vi "test14.2-MappingRelationshipByExternalRegistration_State.vi"() -> ()   [LabVIEW 2017, in "testcase-CSMBroadcast.lvclass"]
uses:
  testcase-CSMBroadcast.lvclass
  5f1321ef-d679-4204-8b32-271554a776bf.vi
  3afc563d-56e9-48a4-901d-19be23a22e68.vi
  src/user.lib/_NEVSTOP/Communicable State Machine(CSM)/AdvanceAPI/CSM - Revert Arguments-Safe String.vi
  src/user.lib/_NEVSTOP/Communicable State Machine(CSM)/AdvanceAPI/CSM - Make String Arguments Safe.vi
  src/user.lib/_NEVSTOP/Communicable State Machine(CSM)/AdvanceAPI/CSM - Break Down Multiple States String.vi
  src/user.lib/_NEVSTOP/Communicable State Machine(CSM)/AdvanceAPI/CSM - Keywords.vi
  src/user.lib/_NEVSTOP/Communicable State Machine(CSM)/_Polymophic/CSM - Replace Marks in Messages.vi
  src/user.lib/_NEVSTOP/Communicable State Machine(CSM)/_Shared/Trim Single-line Text.vi
  src/user.lib/_NEVSTOP/Communicable State Machine(CSM)/Communicable State Machine.lvlib
  <vilib>/addons/_JKI Toolkits/VI Tester/TestCase.llb/TestCase.lvclass
  CSM/CSM-Testcase.lvlib
  C:/Program Files (x86)/National Instruments/LabVIEW 2017/vi.lib/addons/_JKI Toolkits/VI Tester/TestCase.llb/TestCase.lvclass
panel:
  out "State History 2":string
  out "Loop Count":i32
  out "TestCase out":refnum<class "testcase-CSMBroadcast.lvclass">
  in  "TestCase in":refnum<class "testcase-CSMBroadcast.lvclass">
  out "error out":errorcluster
  in  "error in (no error)":errorcluster
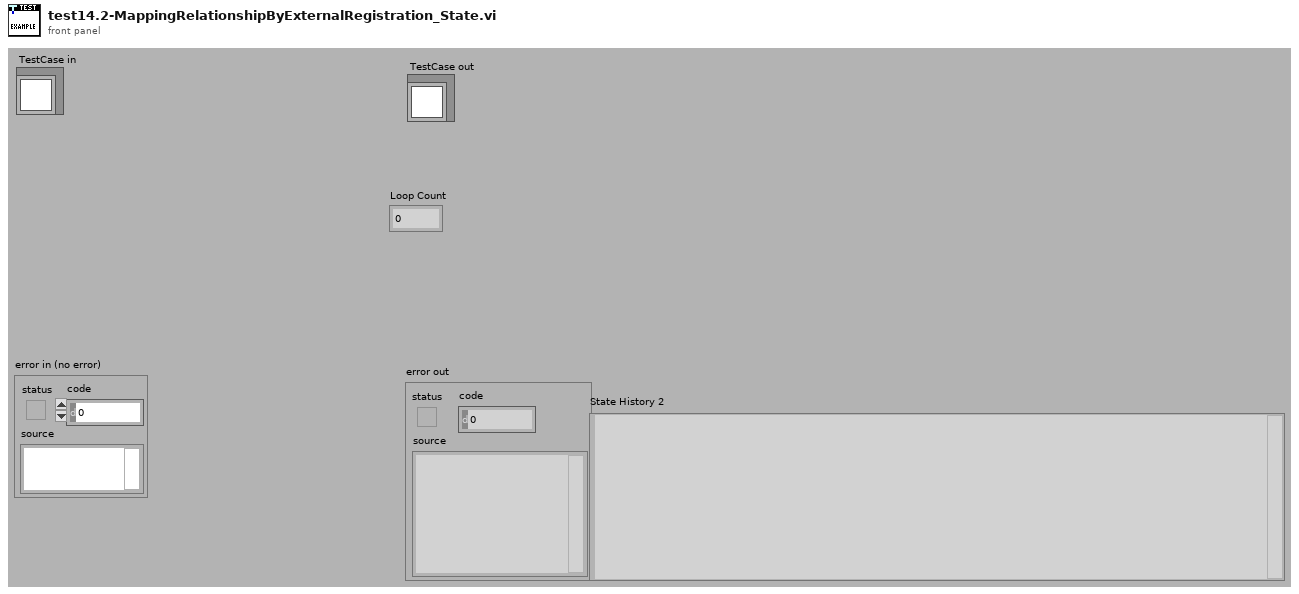
[diagram p1: front panel]
types:
  T1 = enum32{"Invalid", "Standard", "Closed", "Hidden", "Minimized", "Maximized"}
  T2 = enum32{"invalid app kind", "Development System", "Run Time System", "Student Edition", "Embedded LabVIEW", "Evaluation", "Custom"}
  T3 = cluster{"Status":string, "Source CSM":string, "Target CSM":string, "Target API":string}[]
  T4 = typedef "Communicable State Machine.lvlib/_CSM_Response Source Message.ctl" = cluster{"‘State":string, "’Arguments":string, "’Error":errorcluster}
  T5 = cluster{"Current VI Reference":refnum<vi>, "Close Panel on Exit?":bool}
  T6 = cluster{"Core":cluster{"Current VI Reference":refnum<vi>, "Close Panel on Exit?":bool}, "Your Boolean data":bool, "Your string data":string}
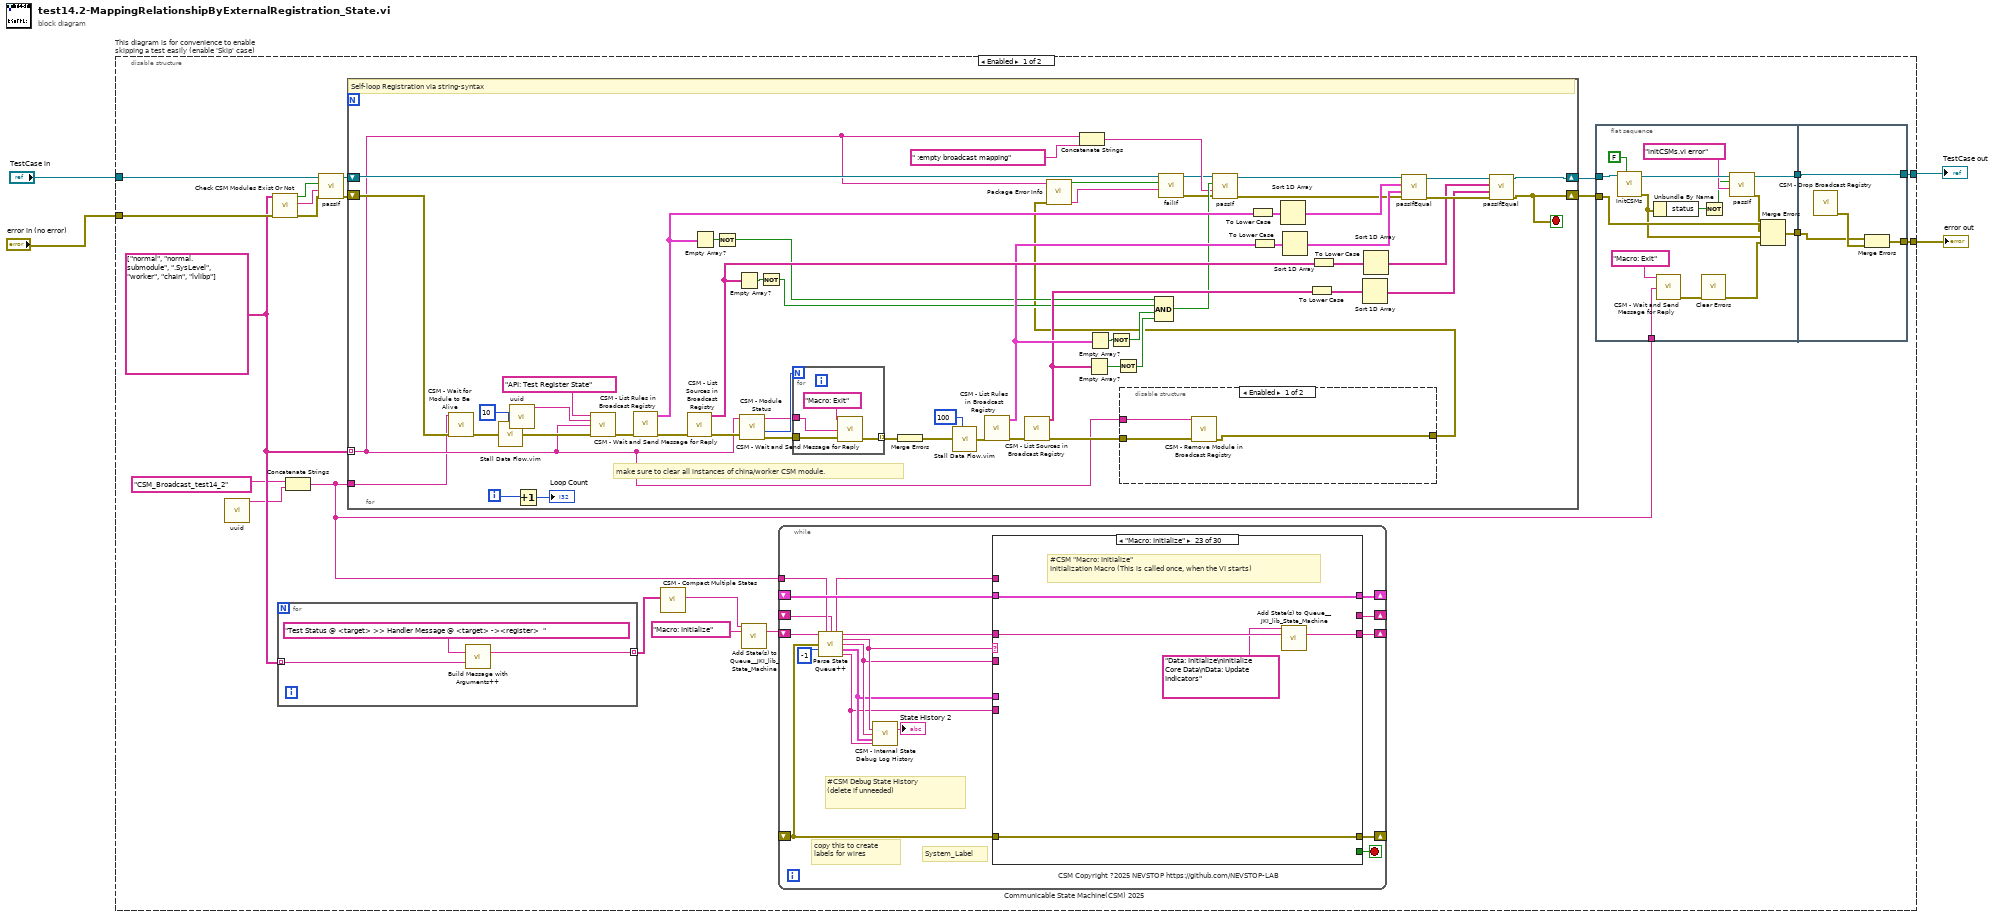
[diagram p0: block diagram]
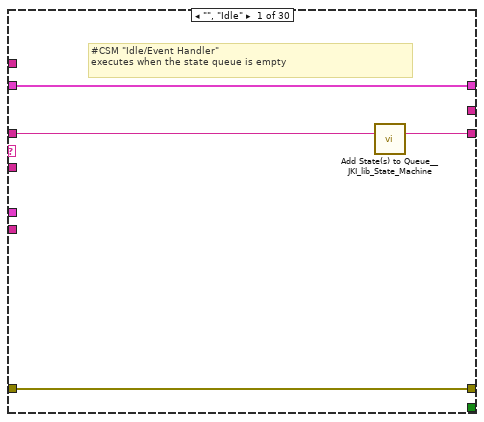
[diagram p2: hidden frame]
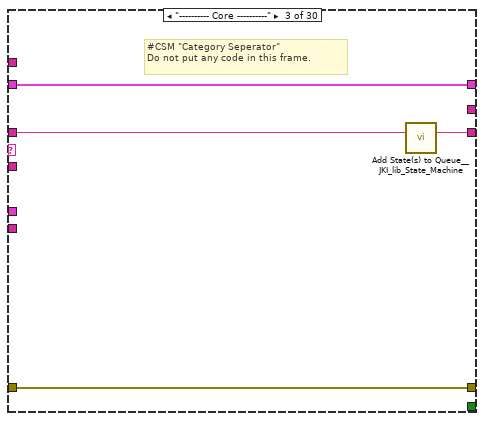
[diagram p4: hidden frame]
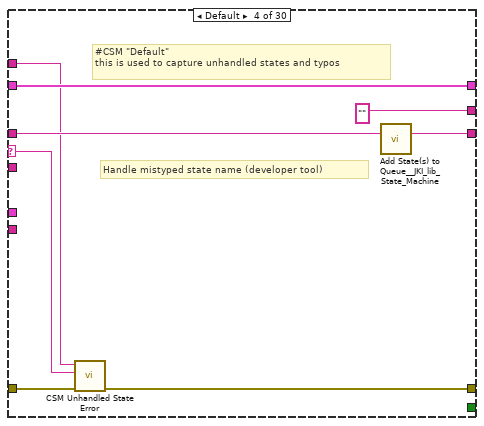
[diagram p5: hidden frame]
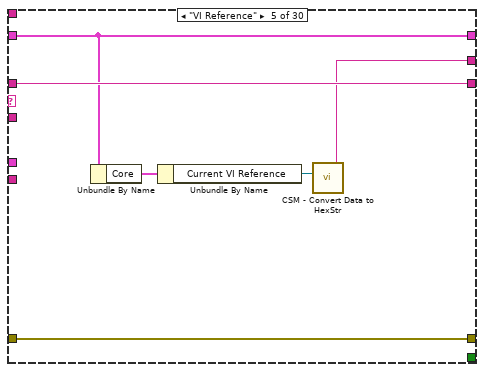
[diagram p6: hidden frame]
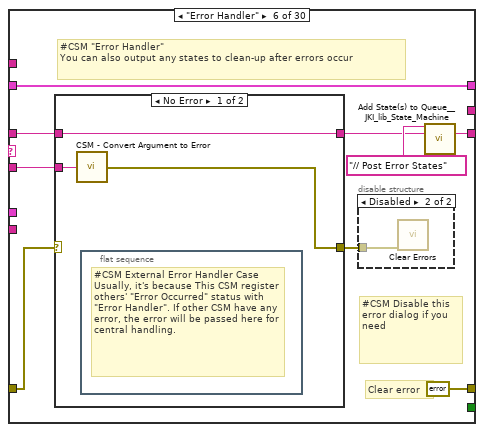
[diagram p7: hidden frame]
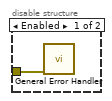
[diagram p8: hidden frame]
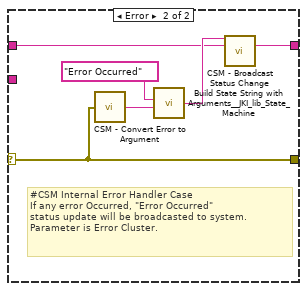
[diagram p9: hidden frame]
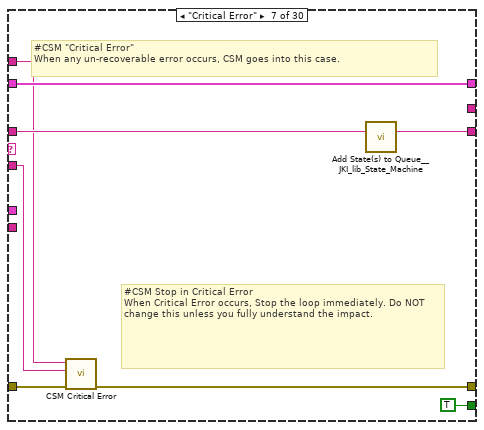
[diagram p10: hidden frame]
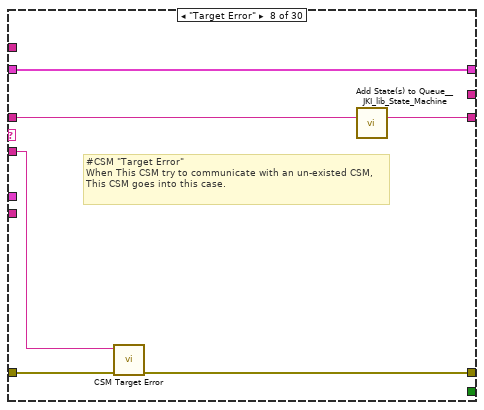
[diagram p11: hidden frame]
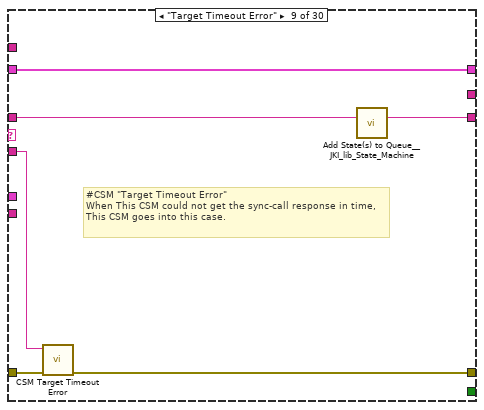
[diagram p12: hidden frame]
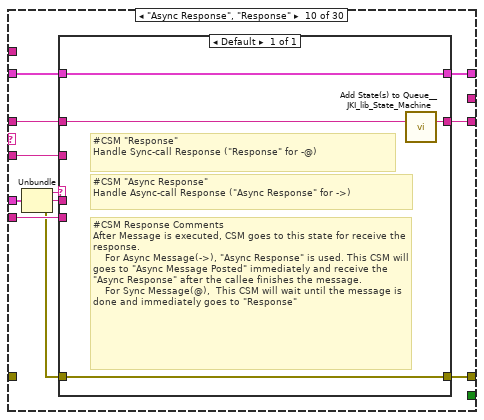
[diagram p13: hidden frame]
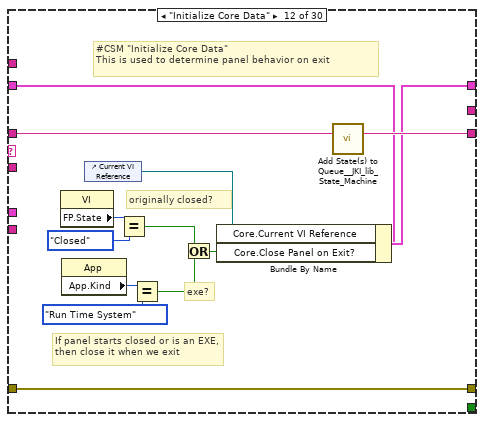
[diagram p15: hidden frame]
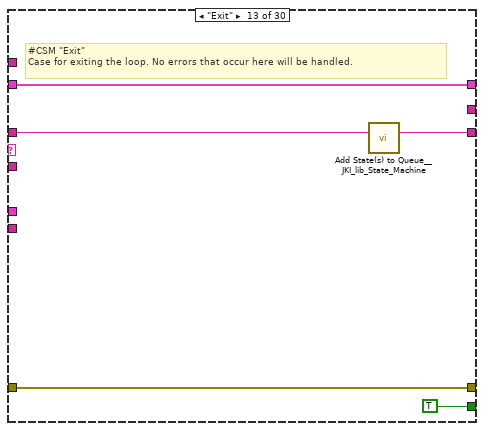
[diagram p16: hidden frame]
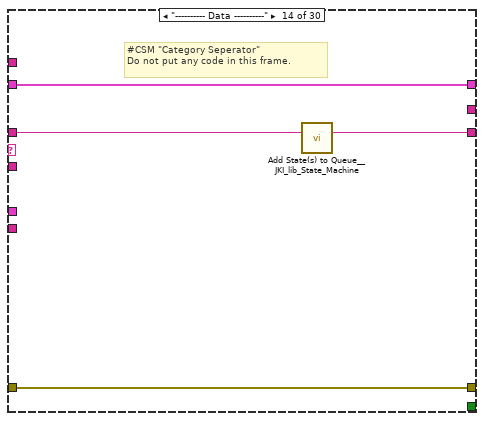
[diagram p17: hidden frame]
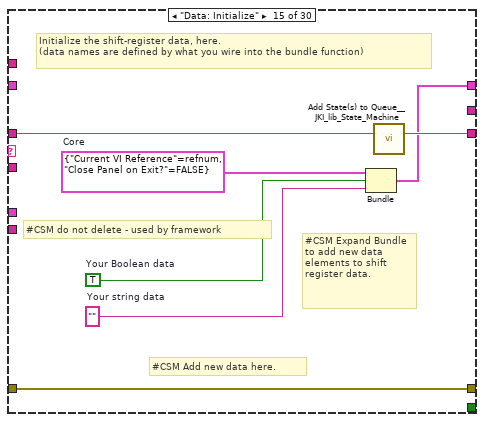
[diagram p18: hidden frame]
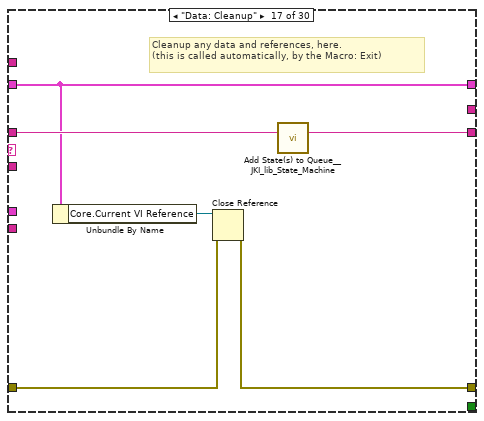
[diagram p20: hidden frame]
diagram:
  n1 = disable-structure "This diagram is for convenience to enable skipping a test easily (enable 'Skip' case)" shown="Enabled" {
    disable-tunnel: "TestCase in" -> [w20 w401]
    disable-tunnel: [w14 w399] -> w1
    disable-tunnel: [w13 w400] -> w3
    disable-tunnel: "error in (no error)" -> [w22 w398]
    frame Enabled {
      w10 = string[] ["normal", "normal.submodule", ".SysLevel", "worker", "chain", "lvlibp"]
      n2 = call "uuid.vi"() -> ("UUID"=w6:string)  [unwired: 11 in]
      n3 = call "Check CSM Modules Exist Or Not.vi"("error in"=w22, "CSM names in"=w10) -> ("error out"=w23:errorcluster, "Debug string"=w24:string, "All Modules Exist?"=w25:bool)  [unwired: 7 in]
      n4 = for {
        tunnel: w10 -> [w27] mode=indexing
        tunnel: [w26] -> w9 mode=indexing
        n5 = call-poly "Build Message with Arguments++.vi"("States With Replace Token"="Test Status @ <target> >> Handler Message @ <target> -><register>  " ("State"), "<target>"=w27) -> ("States"=w26:string)  [unwired: 13 in]
      }
      n6 = Concatenate Strings("CSM_Broadcast_test14_2" ("Name (\"\" to Use UUID)"), w6) -> (w5:string)
      n7 = call-dynamic "passIf.vi"("error in (no error)"=w23, "message (\"\")"=w24, "pass"=w25, "TestCase in"=w20) -> ("error out"=w21:errorcluster, "TestCase out"=w19:refnum<class "testcase-CSMBroadcast.lvclass">)  [unwired: 6 in]
      n8 = for {
        tunnel: w10 -> [w329] mode=indexing
        shift-right: [w324] -> w16
        shift-left: w19 -> [w334]
        shift-right: [w323] -> w15
        shift-left: w21 -> [w340]
        tunnel: w5 -> [w326]
        i -> [w363]
        stop <- w323 stop-if-true
        # "make sure to clear all instances of china/worker CSM module."
        # "Self-loop Registration via string-syntax"
        n9 = call "CSM - Wait for Module to Be Alive.vi"("CSM Name"=w326, "error in (no error)"=w340) -> ("error out"=w348:errorcluster)  [unwired: 11 in, 2 out]
        n10 = call "Stall Data Flow.vim"("value in"=w348, "milliseconds to wait"=u32 10) -> ("value out"=w347:errorcluster)  [unwired: 1 out]
        n11 = call "uuid.vi"() -> ("UUID"=w378:string)  [unwired: 11 in]
        n12 = Increment(x=w363) -> (x+1=→"Loop Count":i32)
        n13 = call "CSM - Wait and Send Message for Reply.vi"("State"="API: Test Register State", "Arguments (\"\")"=w378, "Target Module"=w329, "Error In (No Error)"=w347) -> ("error out"=w377:errorcluster)  [unwired: 8 in, 3 out]
        n14 = call "CSM - List Rules in Broadcast Registry.vi"("error in (no error)"=w377) -> ("error out"=w375:errorcluster, "Rule Entries"=w361:T3)  [unwired: 8 in, 1 out]
        n15 = call "CSM - List Sources in Broadcast Registry.vi"("error in (no error)"=w375) -> ("error out"=w342:errorcluster, "Broadcast Names"=w358:string[])  [unwired: 9 in]
        n16 = Empty Array?(array=w361) -> (empty?=w360:bool)
        n17 = Not(x=w360) -> (.not. x?=w353:bool)
        n18 = Empty Array?(array=w358) -> (empty?=w359:bool)
        n19 = call "CSM - Module Status.vi"("Error In"=w342, "CSM Name"=w329) -> ("error out"=w343:errorcluster, "#Nodes"=w345:i32, "CSM Name (Dup)"=w344:string)  [unwired: 5 in, 2 out]
        n20 = Not(x=w359) -> (.not. x?=w352:bool)
        n21 = for {
          N: w345 -> [_]
          tunnel: w344 -> [w382]
          tunnel: w343 -> [w380]
          tunnel: [w381] -> w376 mode=indexing
          n22 = call "CSM - Wait and Send Message for Reply.vi"("State"="Macro: Exit", "Target Module"=w382, "Error In (No Error)"=w380) -> ("error out"=w381:errorcluster)  [unwired: 9 in, 3 out]
        }
        n23 = Merge Errors(w376) -> (w331:errorcluster)
        n24 = call "Stall Data Flow.vim"("value in"=w331, "milliseconds to wait"=u32 100) -> ("value out"=w330:errorcluster)  [unwired: 1 out]
        n25 = call "CSM - List Rules in Broadcast Registry.vi"("error in (no error)"=w330) -> ("error out"=w374:errorcluster, "Rule Entries"=w356:T3)  [unwired: 8 in, 1 out]
        n26 = call "CSM - List Sources in Broadcast Registry.vi"("error in (no error)"=w374) -> ("error out"=w351:errorcluster, "Broadcast Names"=w354:string[])  [unwired: 9 in]
        n27 = Concatenate Strings(w329, " :empty broadcast mapping" ("string")) -> (w336:string)
        n28 = Empty Array?(array=w354) -> (empty?=w355:bool)
        n29 = Empty Array?(array=w356) -> (empty?=w357:bool)
        n30 = Not(x=w357) -> (.not. x?=w350:bool)
        n31 = Not(x=w355) -> (.not. x?=w349:bool)
        n32 = disable-structure shown="Enabled" {
          disable-tunnel: w351 -> [w386 w390]
          disable-tunnel: w329 -> [w385 w391]
          disable-tunnel: [w384 w389] -> w325
          frame Enabled {
            n33 = call "CSM - Remove Module in Broadcast Registry.vi"("CSM Name"=w385, "Error In"=w386) -> ("error out"=w384:errorcluster)  [unwired: 12 in, 1 out]
          }
          frame Disabled {
            n34 = flat-sequence {
              tunnel: "Test Status" ("Status") -> [w397]
              tunnel: "Handler Message" ("Response Message (If \"\", Same as Source Message)") -> [w396]
              tunnel: w391 -> [w395]
              tunnel: w390 -> [w394]
              tunnel: [w392] -> w389
              frame #0 {
                n35 = call "CSM - Unregister Broadcast.vi"("CSM Name(Empty for Broadcast Event)"=w395, "Source CSM Name (* as Default)"=w395, "Trigger"=w397, "API (\"*\" as Default)"=w396) -> ("error out"=w393:errorcluster)  [unwired: 10 in, 1 out]
                n36 = Merge Errors(w394, w393) -> (w392:errorcluster)
              }
            }
          }
        }
        n37 = call "Package Error Info.vi"("error in"=w325, "String in"=w329) -> ("packed error info out"=w327:string, "error status"=w328:bool)  [unwired: 8 in]
        n38 = Compound Arithmetic op=AND(w353, w352, w350, w349) -> (w338:bool)
        n39 = call-dynamic "failIf.vi"("message (\"\")"=w327, "fail"=w328, "TestCase in"=w334) -> ("error out"=w333:errorcluster, "TestCase out"=w335:refnum<class "testcase-CSMBroadcast.lvclass">)  [unwired: 7 in]
        n40 = call-dynamic "passIf.vi"("error in (no error)"=w333, "message (\"\")"=w336, "pass"=w338, "TestCase in"=w335) -> ("error out"=w339:errorcluster, "TestCase out"=w341:refnum<class "testcase-CSMBroadcast.lvclass">)  [unwired: 6 in]
        n41 = To Lower Case(string=w361) -> (all lower case string=w373:T3)
        n42 = To Lower Case(string=w356) -> (all lower case string=w372:T3)
        n43 = Sort 1D Array(array=w373) -> (sorted array=w371:T3)
        n44 = Sort 1D Array(array=w372) -> (sorted array=w370:T3)
        n45 = To Lower Case(string=w354) -> (all lower case string=w366:string[])
        n46 = To Lower Case(string=w358) -> (all lower case string=w367:string[])
        n47 = Sort 1D Array(array=w366) -> (sorted array=w364:string[])
        n48 = Sort 1D Array(array=w367) -> (sorted array=w365:string[])
        n49 = call-dynamic "passIfEqual.vi"("error in (no error)"=w339, "y"=w370, "x"=w371, "TestCase in"=w341) -> ("error out"=w368:errorcluster, "TestCase out"=w369:refnum<class "testcase-CSMBroadcast.lvclass">)  [unwired: 6 in]
        n50 = call-dynamic "passIfEqual.vi"("error in (no error)"=w368, "y"=w364, "x"=w365, "TestCase in"=w369) -> ("error out"=w323:errorcluster, "TestCase out"=w324:refnum<class "testcase-CSMBroadcast.lvclass">)  [unwired: 6 in]
      }
      n51 = call "CSM - Compact Multiple States.vi"("Multiple States"=w9) -> ("States"=w8:string)  [unwired: 9 in]
      n52 = call <vilib>:"Add State(s) to Queue__JKI_lib_State_Machine.vi"("State(s) in Front (\"\")"=w8, "State(s) in (\"\")"="Macro: Initialize" ("Init State(\"Macro: Initialize\")")) -> ("States Out"=w11:string)  [unwired: 13 in]
      n53 = while "Communicable State Machine(CSM) 2025" {
        shift-right: [w41] -> _
        shift-left: _ -> [w40]
        shift-right: [w44] -> _
        shift-left: _ -> [w39]
        shift-right: [w43] -> _
        shift-left: w11 -> [w45]
        tunnel: w5 -> [w37]
        shift-right: [w38] -> _
        shift-left: _ -> [w31]
        stop <- w42 stop-if-true
        # "#CSM Debug State History\n(delete if unneeded)"
        # "copy this to create labels for wires"
        # "System_Label"
        # "CSM Copyright ?2025 NEVSTOP https://github.com/NEVSTOP-LAB"
        n54 = call "Parse State Queue++.vi"("State Queue"=w45, "Name (\"\" to Use UUID)"=w37, "Response Arguments"=w31, "Previous Error"=w39, "Dequeue (1 ms)"=-1 ("Timeout")) -> ("Name Used"=w32:string, "Remaining States"=w46:string, "Current State"=w36:string, "Arguments"=w35:string, "Additional Information"=w34:T4, "Source CSM"=w33:string)  [unwired: 5 in]
        n55 = call "CSM - Internal State Debug Log History.vi"("State"=w36, "Arguments (\"\")"=w35, ">> Response Source Message >>"=w34, "Source (\"\")"=w33) -> ("Debug Log"=→"State History 2":string)  [unwired: 11 in]
        n56 = case shown="\"Macro: Initialize\"" w36 {
          selector: w36 -> [_ _ _ w60 _ _ _ _ _ _ _ _ _ _ _ _ _ _ _ _ _ _ _ _ _ _ _ _ _ _]
          tunnel: w46 -> [w47 w52 w57 w64 w70 w76 w97 w103 w109 w117 w128 w142 w147 w151 w158 w160 w167 w171 w175 w181 w196 w265 w270 w277 w279 w283 w288 w295 w299 w303]
          tunnel: w35 -> [_ _ _ _ _ w75 w93 w102 w107 w116 _ _ _ _ _ _ _ _ _ w176 w190 _ _ _ _ _ w286 _ _ _]
          tunnel: w40 -> [w48 w51 w54 w62 w69 w79 w98 w104 w110 w119 w127 w135 w145 w148 _ w159 w162 w168 w173 w179 w192 w262 w267 w274 w278 w282 w287 w292 w296 w300]
          tunnel: [w49 w53 w55 w58 w71 errorcluster {"status"=FALSE, "code"=0, "source"=""} ("error out") w94 w100 w106 w122 w129 w139 w144 w149 w155 w161 w163 w169 w172 w177 w193 w263 w268 w275 w280 w284 w289 w293 w297 w301] -> w44
          tunnel: w39 -> [w49 w53 w55 w65 w71 w77 w99 w101 w108 _ w129 w139 w144 w149 w155 w161 w164 w169 w172 w178 w194 w263 w268 w275 w280 w284 w289 w293 w297 w301]
          tunnel: [w50 w52 w56 w63 w70 w72 w96 w105 w111 w118 w128 w141 w146 w150 w157 w160 w166 w170 w174 w180 w195 w264 w269 w276 w279 w283 w288 w294 w298 w302] -> w43
          tunnel: [_ _ _ _ _ _ TRUE _ _ _ _ _ TRUE _ _ _ _ _ _ _ _ _ _ _ _ _ _ _ _ _] -> w42
          tunnel: [w48 w51 w54 w62 w69 w79 w98 w104 w110 w120 w127 w140 w145 w148 w156 w159 w162 w168 w173 w179 w192 w262 w267 w274 w278 w282 w287 w292 w296 w300] -> w41
          tunnel: w33 -> [_ _ _ _ _ _ _ _ _ w114 _ _ _ _ _ _ _ _ _ _ _ _ _ _ _ _ _ _ _ _]
          tunnel: w34 -> [_ _ _ _ _ _ _ _ _ w121 _ _ _ _ _ _ _ _ _ _ _ _ _ _ _ _ _ _ _ _]
          tunnel: [_ _ _ "" w66 _ _ _ _ _ _ _ _ _ _ _ _ _ _ _ _ _ _ _ _ "API1 Response" w285 _ _ _] -> w38
          tunnel: w32 -> [_ _ _ w59 _ _ w92 _ _ _ _ _ _ _ _ _ _ _ _ _ _ _ _ _ _ _ _ _ _ _]
          frame "", "Idle" {
            # "#CSM \"Idle/Event Handler\"\nexecutes when the state queue is empty"
            n57 = call <vilib>:"Add State(s) to Queue__JKI_lib_State_Machine.vi"("State(s) in (\"\")"=w47) -> ("States Out"=w50:string)  [unwired: 14 in]
          }
          frame "CSM Documentation" {
            # "#CSM README FIRST\n\nCommunicable State Machine(CSM) is a LabVIEW application framework that builds upon JKI State Machine(JKISM). It follows the pattern of JKISM and extends the keywords to describe message communication between modules, including concepts such as Sync-Message, Async-Message, Subscription/Unsubscription of status - essential elements for creating reusable code modules. For more information, please visit the CSM wiki: https://nevstop-lab.github.io/CSM-Wiki/\n\nFor instructions on JKI State Machine, visit: http://jki.net/state-machine/\nFor information about CSM, visit: https://github.com/NEVSTOP-LAB"
            # "#CSM \"Documentation\"\nCase for holding CSM Documenation"
          }
          frame "---------- Core ----------" {
            # "#CSM \"Category Seperator\"\nDo not put any code in this frame."
            n58 = call <vilib>:"Add State(s) to Queue__JKI_lib_State_Machine.vi"("State(s) in (\"\")"=w57) -> ("States Out"=w56:string)  [unwired: 14 in]
          }
          frame Default {
            # "#CSM \"Default\"\nthis is used to capture unhandled states and typos"
            # "Handle mistyped state name (developer tool)"
            n59 = call "CSM Unhandled State Error.vi"("error in (no error)"=w65, "Undefined State"=w60, "CSM Name"=w59) -> ("error out"=w58:errorcluster)  [unwired: 8 in]
            n60 = call <vilib>:"Add State(s) to Queue__JKI_lib_State_Machine.vi"("State(s) in (\"\")"=w64) -> ("States Out"=w63:string)  [unwired: 14 in]
          }
          frame "VI Reference" {
            n61 = Unbundle By Name(w69) -> ("Core"=w68:T5)
            n62 = Unbundle By Name(w68) -> ("Current VI Reference"=w67:refnum<vi>)
            n63 = call "CSM - Convert Data to HexStr.vi"("Variant"=w67) -> ("HEX String (0-9,A-F)"=w66:string)  [unwired: 8 in]
          }
          frame "Error Handler" {
            # "#CSM Disable this error dialog if you need"
            # "#CSM \"Error Handler\"\nYou can also output any states to clean-up after errors occur"
            # "Clear error"
            n64 = case shown="No Error" w77 {
              selector: w77 -> [_ w86]
              tunnel: [w85 w88] -> w73
              tunnel: w76 -> [w85 w87]
              tunnel: w75 -> [w84 _]
              tunnel: [w83 w86] -> w78
              frame No Error {
                n65 = call "CSM - Convert Argument to Error.vi"("Argument"=w84) -> ("Error"=w83:errorcluster)  [unwired: 4 in]
                n66 = flat-sequence {
                  frame #0 {
                    # "#CSM External Error Handler Case\nUsually, it's because This CSM register others' \"Error Occurred\" status with \"Error Handler\". If other CSM have any error, the error will be passed here for central handling."
                  }
                }
              }
              frame Error {
                # "#CSM Internal Error Handler Case \nIf any error Occurred, \"Error Occurred\" \nstatus update will be broadcasted to system.\nParameter is Error Cluster."
                n67 = call "CSM - Convert Error to Argument.vi"("Error"=w86) -> ("Argument"=w90:string)  [unwired: 4 in]
                n68 = call <vilib>:"Build State String with Arguments__JKI_lib_State_Machine.vi"("Arguments (\"\")"=w90, "State"="Error Occurred" ("Status with Arguments")) -> ("State with Arguments"=w89:string)  [unwired: 4 in]
                n69 = call "CSM - Broadcast Status Change.vi"("Status With Arguments"=w89, "State Queue"=w87) -> ("Remaining States"=w88:string)  [unwired: 13 in]
              }
            }
            n70 = disable-structure shown="Disabled" {
              disable-tunnel: w78 -> [w81 w82]
              frame Enabled {
                n71 = call <vilib>:"General Error Handler.vi"("error in (no error)"=w81) -> ()  [unwired: 10 in, 5 out]
              }
              frame Disabled {
                n72 = call <vilib>:"Clear Errors.vi"("error in (no error)"=w82) -> ()  [unwired: 5 in, 2 out]
              }
            }
            n73 = call <vilib>:"Add State(s) to Queue__JKI_lib_State_Machine.vi"("State(s) in Front (\"\")"="// Post Error States", "State(s) in (\"\")"=w73) -> ("States Out"=w72:string)  [unwired: 13 in]
          }
          frame "Critical Error" {
            # "#CSM Stop in Critical Error\nWhen Critical Error occurs, Stop the loop immediately. Do NOT change this unless you fully understand the impact."
            # "#CSM \"Critical Error\"\nWhen any un-recoverable error occurs, CSM goes into this case."
            n74 = call "CSM Critical Error.vi"("error in (no error)"=w99, "Arugments (As Reason)"=w93, "CSM Name"=w92) -> ("error out"=w94:errorcluster)  [unwired: 8 in]
            n75 = call <vilib>:"Add State(s) to Queue__JKI_lib_State_Machine.vi"("State(s) in (\"\")"=w97) -> ("States Out"=w96:string)  [unwired: 14 in]
          }
          frame "Target Error" {
            # "#CSM \"Target Error\"\nWhen This CSM try to communicate with an un-existed CSM, This CSM goes into this case."
            n76 = call "CSM Target Error.vi"("error in (no error)"=w101, "Arguments (As CSM Name)"=w102) -> ("error out"=w100:errorcluster)  [unwired: 9 in]
            n77 = call <vilib>:"Add State(s) to Queue__JKI_lib_State_Machine.vi"("State(s) in (\"\")"=w103) -> ("States Out"=w105:string)  [unwired: 14 in]
          }
          frame "Target Timeout Error" {
            # "#CSM \"Target Timeout Error\"\nWhen This CSM could not get the sync-call response in time, This CSM goes into this case."
            n78 = call "CSM Target Timeout Error.vi"("error in (no error)"=w108, "Arguments (As CSM Name)"=w107) -> ("error out"=w106:errorcluster)  [unwired: 9 in]
            n79 = call <vilib>:"Add State(s) to Queue__JKI_lib_State_Machine.vi"("State(s) in (\"\")"=w109) -> ("States Out"=w111:string)  [unwired: 14 in]
          }
          frame "Async Response", "Response" {
            n80 = Unbundle(w121) -> ("‘State"=w115:string, "’Arguments"=w113:string, "’Error"=w112:errorcluster)
            n81 = case shown="Default" w115 {
              tunnel: [w126] -> w122
              tunnel: w112 -> [w126]
              tunnel: [w125] -> w120
              tunnel: w119 -> [w125]
              tunnel: [w123] -> w118
              tunnel: w117 -> [w124]
              tunnel: w116 -> [_]
              tunnel: w114 -> [_]
              tunnel: w113 -> [_]
              frame Default {
                # "#CSM Response Comments\nAfter Message is executed, CSM goes to this state for receive the response.\n    For Async Message(->), \"Async Response\" is used. This CSM will goes to \"Async Message Posted\" immediately and receive the \"Async Response\" after the callee finishes the message.\n    For Sync Message(@),  This CSM will wait until the message is done and immediately goes to \"Response\""
                # "#CSM \"Async Response\"\nHandle Async-call Response (\"Async Response\" for ->)"
                # "#CSM \"Response\"\nHandle Sync-call Response (\"Response\" for -@)"
                n82 = call <vilib>:"Add State(s) to Queue__JKI_lib_State_Machine.vi"("State(s) in (\"\")"=w124) -> ("States Out"=w123:string)  [unwired: 14 in]
              }
            }
          }
          frame "Async Message Posted" {
            # "#CSM \"Async Message Posted\"\nAfter Async Message is posted (-> or ->| ), CSM goes to this state for post-action.\nYou can use Argument - State to tell which Async Message is called."
          }
          frame "Initialize Core Data" {
            # "#CSM \"Initialize Core Data\"\nThis is used to determine panel behavior on exit"
            # "originally closed?"
            # "exe?"
            # "If panel starts closed or is an EXE, then close it when we exit"
            n83 = property class="VI"() -> ("FP.State"=w132:T1)  [unwired: 2 in, 2 out]
            n84 = property class="App"() -> ("App.Kind"=w138:T2)  [unwired: 2 in, 2 out]
            n85 = control-ref of="Current VI Reference"() -> (w133:refnum<vi>)
            n86 = Equal?(x=w132, y=T1."Closed" ("Front Panel Window:State")) -> (x = y?=w130:bool)
            n87 = Equal?(x=w138, y=T2."Run Time System" ("Application:Kind")) -> (x = y?=w136:bool)
            n88 = Or(x=w130, y=w136) -> (x .or. y?=w134:bool)
            n89 = Bundle By Name(cluster=w135, "Core.Current VI Reference"=w133, "Core.Close Panel on Exit?"=w134) -> (w140:T6)
            n90 = call <vilib>:"Add State(s) to Queue__JKI_lib_State_Machine.vi"("State(s) in (\"\")"=w142) -> ("States Out"=w141:string)  [unwired: 14 in]
          }
          frame "Exit" {
            # "#CSM \"Exit\"\nCase for exiting the loop. No errors that occur here will be handled."
            n91 = call <vilib>:"Add State(s) to Queue__JKI_lib_State_Machine.vi"("State(s) in (\"\")"=w147) -> ("States Out"=w146:string)  [unwired: 14 in]
          }
          frame "---------- Data ----------" {
            # "#CSM \"Category Seperator\"\nDo not put any code in this frame."
            n92 = call <vilib>:"Add State(s) to Queue__JKI_lib_State_Machine.vi"("State(s) in (\"\")"=w151) -> ("States Out"=w150:string)  [unwired: 14 in]
          }
          frame "Data: Initialize" {
            w152 = T5 {"Current VI Reference"=refnum, "Close Panel on Exit?"=FALSE}  # Core
            w154 = TRUE  # Your Boolean data
            w153 = ""  # Your string data
            # "#CSM do not delete - used by framework"
            # "#CSM Expand Bundle to add new data elements to shift register data."
            # "#CSM Add new data here."
            # "Initialize the shift-register data, here.\n(data names are defined by what you wire into the bundle function)"
            n93 = Bundle("Core"=w152, "Your Boolean data"=w154, "Your string data"=w153) -> (w156:T6)  [unwired: 1 in]
            n94 = call <vilib>:"Add State(s) to Queue__JKI_lib_State_Machine.vi"("State(s) in (\"\")"=w158) -> ("States Out"=w157:string)  [unwired: 14 in]
          }
          frame "Data: Update Indicators" {
          }
          frame "Data: Cleanup" {
            # "Cleanup any data and references, here.\n(this is called automatically, by the Macro: Exit)"
            n95 = Unbundle By Name(w162) -> ("Core.Current VI Reference"=w165:refnum<vi>)
            n96 = Close Reference(reference=w165, error in (no error)=w164) -> (error out=w163:errorcluster)
            n97 = call <vilib>:"Add State(s) to Queue__JKI_lib_State_Machine.vi"("State(s) in (\"\")"=w167) -> ("States Out"=w166:string)  [unwired: 14 in]
          }
          frame "---------- UI ----------" {
            # "#CSM \"Category Seperator\"\nDo not put any code in this frame."
            n98 = call <vilib>:"Add State(s) to Queue__JKI_lib_State_Machine.vi"("State(s) in (\"\")"=w171) -> ("States Out"=w170:string)  [unwired: 14 in]
          }
          frame "UI: Initialize" {
            # "#CSM \"UI: Initialize\"\nInitialize the User Interface, here.\n(this is called automatically, by the Macro: Init)"
            n99 = call <vilib>:"Add State(s) to Queue__JKI_lib_State_Machine.vi"("State(s) in (\"\")"=w175) -> ("States Out"=w174:string)  [unwired: 14 in]
          }
          frame "UI: Cursor Set" {
            # "#CSM \"UI: Cursor Set\"\nSet and Unset Cursor Busy.\n(Usage: \"UI: Cursor Set >> Busy|Idle\")"
            # "Argument"
            n100 = disable-structure shown="TARGET_TYPE!=Windows" {
              disable-tunnel: w178 -> [w184 w189]
              disable-tunnel: [w183 w189] -> w177
              disable-tunnel: w176 -> [w182 _]
              frame condition #0 (active) {
                n101 = case shown="\"Idle\", Default" w182 {
                  tunnel: w184 -> [w186 w188]
                  tunnel: [w185 w187] -> w183
                  frame "Idle", Default {
                    n102 = call <vilib>:"Unset Busy.vi"("error in (no error)"=w186) -> ("error out"=w185:errorcluster)  [unwired: 10 in]
                  }
                  frame "Busy" {
                    n103 = call <vilib>:"Set Busy.vi"("error in (no error)"=w188) -> ("error out"=w187:errorcluster)  [unwired: 9 in, 1 out]
                  }
                }
              }
              frame condition #1 {
              }
            }
            n104 = call <vilib>:"Add State(s) to Queue__JKI_lib_State_Machine.vi"("State(s) in (\"\")"=w181) -> ("States Out"=w180:string)  [unwired: 14 in]
          }
          frame "UI: Front Panel State" {
            # "#CSM \"UI: Front Panel State\"\nSet Front Panel Open or Closed\n(Usage: \"UI: Front Panel State >> Open|Close\")"
            # "Argument"
            n105 = Unbundle By Name(w192) -> ("Core.Current VI Reference"=w191:refnum<vi>)
            n106 = call <vilib>:"Add State(s) to Queue__JKI_lib_State_Machine.vi"("State(s) in (\"\")"=w196) -> ("States Out"=w195:string)  [unwired: 14 in]
            n107 = case shown="\"Close\", \"Closed\"" w190 {
              tunnel: w194 -> [w202 w217 w228 w241 w254]
              tunnel: [w204 w218 w230 w243 w256] -> w193
              tunnel: w191 -> [w203 w215 w229 w242 w255]
              frame "Open", "Standard", Default {
                w197 = T1."Standard" ("State")
                n108 = property class="VI"(reference=w203, error in=w202) -> (reference out=w200:refnum<vi>, error out=w201:errorcluster, "FP.State"=w199:T1)
                n109 = Not Equal?(x=w199, y=w197) -> (x != y?=w198:bool)
                n110 = case shown="True" w198 {
                  tunnel: [w208 w210] -> w204
                  tunnel: w201 -> [w207 w210]
                  tunnel: w200 -> [w206 _]
                  tunnel: w197 -> [w205 _]
                  frame True {
                    n111 = invoke class="VI" method="FP.Open"(reference=w206, error in=w207, "Activate"=TRUE, "State"=w205) -> (error out=w208:errorcluster)  [unwired: 1 in, 4 out]
                  }
                  frame False {
                  }
                }
              }
              frame "Close", "Closed" {
                n112 = property class="VI"(reference=w215, error in=w217) -> (reference out=w214:refnum<vi>, error out=w216:errorcluster, "FP.State"=w212:T1)
                n113 = Not Equal?(x=w212, y=T1."Closed" ("Front Panel Window:State")) -> (x != y?=w211:bool)
                n114 = case shown="False" w211 {
                  tunnel: [w219 w222] -> w218
                  tunnel: w216 -> [w219 w221]
                  tunnel: w214 -> [_ w220]
                  frame False {
                  }
                  frame True {
                    n115 = invoke class="VI" method="FP.Close"(reference=w220, error in=w221) -> (error out=w222:errorcluster)  [unwired: 1 in, 2 out]
                  }
                }
              }
              frame "Hidden", "Hide" {
                w223 = T1."Hidden" ("State")
                n116 = property class="VI"(reference=w229, error in=w228) -> (reference out=w226:refnum<vi>, error out=w227:errorcluster, "FP.State"=w225:T1)
                n117 = Not Equal?(x=w225, y=w223) -> (x != y?=w224:bool)
                n118 = case shown="True" w224 {
                  tunnel: [w234 w235] -> w230
                  tunnel: w227 -> [w233 w235]
                  tunnel: w226 -> [w232 _]
                  tunnel: w223 -> [w231 _]
                  frame True {
                    n119 = invoke class="VI" method="FP.Open"(reference=w232, error in=w233, "State"=w231) -> (error out=w234:errorcluster)  [unwired: 2 in, 4 out]
                  }
                  frame False {
                  }
                }
              }
              frame "Minimize", "Minimized" {
                w236 = T1."Minimized" ("State")
                n120 = property class="VI"(reference=w242, error in=w241) -> (reference out=w239:refnum<vi>, error out=w240:errorcluster, "FP.State"=w238:T1)
                n121 = Not Equal?(x=w238, y=w236) -> (x != y?=w237:bool)
                n122 = case shown="True" w237 {
                  tunnel: [w247 w248] -> w243
                  tunnel: w240 -> [w246 w248]
                  tunnel: w239 -> [w245 _]
                  tunnel: w236 -> [w244 _]
                  frame True {
                    n123 = invoke class="VI" method="FP.Open"(reference=w245, error in=w246, "State"=w244) -> (error out=w247:errorcluster)  [unwired: 2 in, 4 out]
                  }
                  frame False {
                  }
                }
              }
              frame "Maximize", "Maximized" {
                w249 = T1."Maximized" ("State")
                n124 = property class="VI"(reference=w255, error in=w254) -> (reference out=w252:refnum<vi>, error out=w253:errorcluster, "FP.State"=w251:T1)
                n125 = Not Equal?(x=w251, y=w249) -> (x != y?=w250:bool)
                n126 = case shown="True" w250 {
                  tunnel: [w260 w261] -> w256
                  tunnel: w253 -> [w259 w261]
                  tunnel: w252 -> [w258 _]
                  tunnel: w249 -> [w257 _]
                  frame True {
                    n127 = invoke class="VI" method="FP.Open"(reference=w258, error in=w259, "State"=w257) -> (error out=w260:errorcluster)  [unwired: 2 in, 4 out]
                  }
                  frame False {
                  }
                }
              }
            }
          }
          frame "---------- Macro ----------" {
            # "#CSM \"Category Seperator\"\nDo not put any code in this frame."
            n128 = call <vilib>:"Add State(s) to Queue__JKI_lib_State_Machine.vi"("State(s) in (\"\")"=w265) -> ("States Out"=w264:string)  [unwired: 14 in]
          }
          frame "Macro: Initialize" {
            # "#CSM \"Macro: Initialize\"\nInitialization Macro (This is called once, when the VI starts)"
            n129 = call <vilib>:"Add State(s) to Queue__JKI_lib_State_Machine.vi"("State(s) in Front (\"\")"="Data: Initialize\nInitialize Core Data\nData: Update Indicators", "State(s) in (\"\")"=w270) -> ("States Out"=w269:string)  [unwired: 13 in]
          }
          frame "Macro: Exit" {
            # "#CSM \"Macro: Exit\"\nExit Macro (This is called once, when the VI exits)"
            n130 = call <vilib>:"Add State(s) to Queue__JKI_lib_State_Machine.vi"("State(s) in Front (\"\")"="//Exit Sub-Modules ", "State(s) at Back (\"\")"="Data: Cleanup\nExit") -> ("States Out"=w272:string)  [unwired: 13 in]
            n131 = call <vilib>:"Add State(s) to Queue__JKI_lib_State_Machine.vi"("State(s) in Front (\"\")"=w272, "State(s) in (\"\")"=w277) -> ("States Out"=w276:string)  [unwired: 13 in]
          }
          frame "---------- API ----------" {
            # "#CSM \"Category Seperator\"\nDo not put any code in this frame."
          }
          frame "API: API1" {
            # "#CSM API Example\nCopy/Rename this case for your own API"
            # "#CSM Response\nConnect this to return the response of your API"
            # "#CSM >> Msg/Rep's CSM >>\nIf you need to tell who triggered this state , use this string. If it's this case itself, this string is \"\"."
            # "#CSM >> Arguments >>\nDeal with the parameter if any"
          }
          frame "API: API2" {
            # "#CSM API Example\nCopy/Rename this case for your own API"
            # "unpack Hex String  to Variant\nif complex parameter is needed."
            n132 = call "CSM - Convert HexStr to Data.vi"("HEX String"=w286) -> ()  [unwired: 7 in, 2 out]
            n133 = disable-structure shown="Disabled" {
              disable-tunnel: [w290 "API2 Response"] -> w285
              frame Disabled {
                # "pack variant to hexstr \nif complex response is needed."
                # "complex Response"
                n134 = call "CSM - Convert Data to HexStr.vi"() -> ("HEX String (0-9,A-F)"=w290:string)  [unwired: 9 in]
              }
              frame Enabled {
              }
            }
          }
          frame "---------- Action ----------" {
            # "#CSM \"Category Seperator\"\nDo not put any code in this frame."
            n135 = call <vilib>:"Add State(s) to Queue__JKI_lib_State_Machine.vi"("State(s) in (\"\")"=w295) -> ("States Out"=w294:string)  [unwired: 14 in]
          }
          frame "Action: action1" {
            # "#CSM \"Internal State\"\nThis category is used for holding internal states"
            n136 = call <vilib>:"Add State(s) to Queue__JKI_lib_State_Machine.vi"("State(s) in (\"\")"=w299) -> ("States Out"=w298:string)  [unwired: 14 in]
          }
          frame "Action: action2" {
            # "#CSM \"Internal State\"\nThis category is used for holding internal states"
            n137 = call <vilib>:"Add State(s) to Queue__JKI_lib_State_Machine.vi"("State(s) in (\"\")"=w303) -> ("States Out"=w302:string)  [unwired: 14 in]
          }
        }
      }
      n138 = flat-sequence {
        tunnel: w16 -> [w318]
        tunnel: [w315] -> w18
        tunnel: w15 -> [w312]
        tunnel: [w309] -> w17
        tunnel: w5 -> [w305]
        tunnel: w18 -> [w321]
        tunnel: [w321] -> w14
        tunnel: [w320] -> w13
        tunnel: w17 -> [w319]
        frame #0 {
          n139 = call "InitCSMs.vi"("Enable building lvlibp?"=FALSE, "testcase-CSMStatus in"=w318) -> ("error out"=w310:errorcluster, "testcase-CSMStatus out"=w316:refnum<class "testcase-CSMBroadcast.lvclass">)  [unwired: 8 in]
          n140 = Unbundle By Name(w310) -> ("status"=w314:bool)
          n141 = call "CSM - Wait and Send Message for Reply.vi"("State"="Macro: Exit", "Target Module"=w305) -> ("error out"=w306:errorcluster)  [unwired: 10 in, 3 out]
          n142 = call <vilib>:"Clear Errors.vi"("error in (no error)"=w306) -> ("error out"=w304:errorcluster)  [unwired: 5 in, 1 out]
          n143 = Not(x=w314) -> (.not. x?=w308:bool)
          n144 = call-dynamic "passIf.vi"("message (\"\")"="initCSMs.vi error" ("message (\"\")"), "pass"=w308, "TestCase in"=w316) -> ("error out"=w311:errorcluster, "TestCase out"=w315:refnum<class "testcase-CSMBroadcast.lvclass">)  [unwired: 7 in]
          n145 = Merge Errors(w312, w311, w310, w304) -> (w309:errorcluster)
        }
        frame #1 {
          n146 = call "CSM - Drop Broadcast Registry.vi"() -> ("error out"=w322:errorcluster)  [unwired: 15 in]
          n147 = Merge Errors(w319, w322) -> (w320:errorcluster)
        }
      }
    }
    frame Disabled {
      # "skip test result while test is under development"
      n148 = call <vilib>:"skip.vi"("error in (no error)"=w398, "TestCase in"=w401) -> ("error out"=w400:errorcluster, "TestCase out"=w399:refnum<class "testcase-CSMBroadcast.lvclass">)  [unwired: 8 in]
    }
  }
  "error out" <- w3
  "TestCase out" <- w1
